vi "Read Exception Status.vi"(8 "error in":errorcluster, 11 "device data model in":refnum<class "Standard Data Model.lvclass">) -> (0 "error out":errorcluster, 2 "exception status":u8, 3 "device data model out":refnum<class "Standard Data Model.lvclass">)   [LabVIEW 2021, in "Standard Data Model.lvclass"]
doc: "Reads any exception status set in the device model. The exeption status is a single 8-bit integer."
uses:
  Standard Data Model.lvclass
  Standard Data Model.lvclass/Standard Data Model.ctl
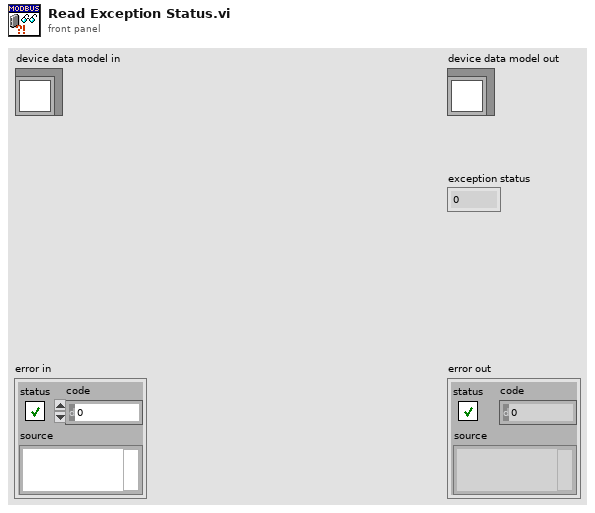
[diagram p1: front panel]
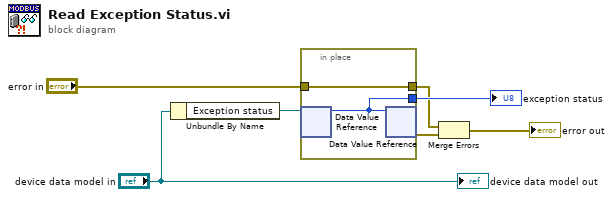
[diagram p0: block diagram]
diagram:
  n1 = Unbundle By Name("device data model in") -> ("Exception status"=w4:refnum<data-value>)
  n2 = in-place {
    in-place-border: "error in" -> [w9]
    in-place-border: [w9] -> w1
    in-place-border: [w8] -> w3
    n3 = in-place-dvr #1(w4) -> (w8:u8)  [unwired: 1 out]
    n4 = in-place-dvr #1(w8) -> (w2:errorcluster)  [unwired: 1 out]
  }
  "exception status" <- w3
  n5 = Merge Errors(w1, w2) -> (→"error out":errorcluster)
  "device data model out" <- "device data model in"
